vi "Execute Example.vi"() -> ()   [LabVIEW 2020]
doc: "This can be used to run a DELETE, INSERT, or UPDATE command. It will return how many rows were affected by the command. It can also be used to execute a query (SELECT statement), but it will not return a result set and the number of affected rows will be -1."
uses:
  <vilib>/Viviota/shared/ORM.lvlibp/ORM/SqlMapper/SqlMapper.lvclass
  <vilib>/Viviota/shared/ORM_DBC_Mssql.lvlibp/DBC.lvclass
panel:
  out "affectedRows":i32
  in  "sqlQuery":string
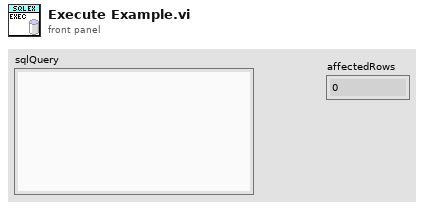
[diagram p1: front panel]
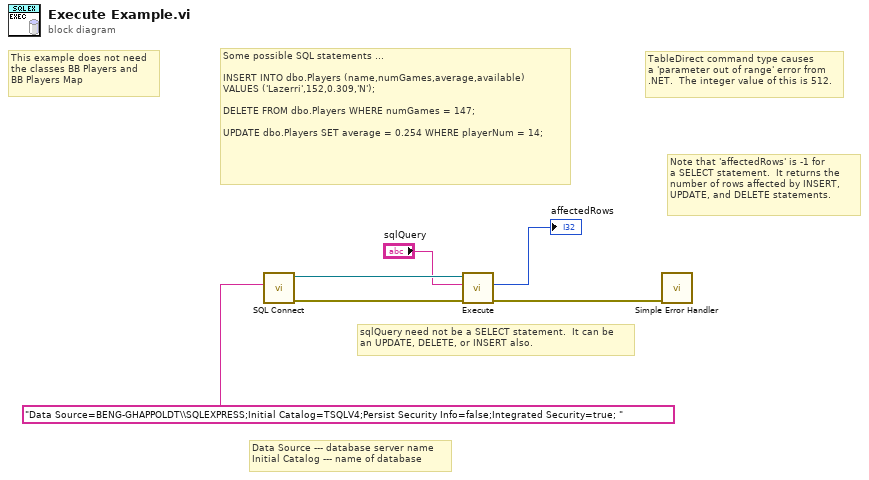
[diagram p0: block diagram]
diagram:
  # "This example does not need\nthe classes BB Players and\nBB Players Map"
  # "sqlQuery need not be a SELECT statement.  It can be\nan UPDATE, DELETE, or INSERT also."
  # "Note that 'affectedRows' is -1 for\na SELECT statement.  It returns the\nnumber of rows affected by INSERT,\nUPDATE, and DELETE statements."
  # "TableDirect command type causes\na 'parameter out of range' error from\n.NET.  The integer value of this is 512."
  # "Some possible SQL statements ...\n\nINSERT INTO dbo.Players (name,numGames,average,available) \nVALUES ('Lazerri',152,0.309,'N');\n\nDELETE FROM dbo.Players WHERE numGames = 147;\n\nUPDATE dbo.Players SET average = 0.254 WHERE playerNum = 14;"
  # "Data Source --- database server name\nInitial Catalog --- name of database"
  n1 = call <vilib>:"SQL Connect.vi"("Connection String"="Data Source=BENG-GHAPPOLDT\\SQLEXPRESS;Initial Catalog=TSQLV4;Persist Security Info=false;Integrated Security=true; ") -> ("error out"=w6:errorcluster, "SQL Mapper"=w4:refnum<class "SqlMapper.lvclass">)  [unwired: 9 in]
  n2 = call-dynamic "Execute.vi"("error in (no error)"=w6, "sql"="sqlQuery", "SqlMapper in"=w4) -> ("error out"=w5:errorcluster, "affectedRows"=→"affectedRows":i32)  [unwired: 6 in, 1 out]
  n3 = call <vilib>:"Simple Error Handler.vi"("error in (no error)"=w5) -> ()  [unwired: 4 in, 5 out]
